vi "Create Segmented Mask.vi"(0 "Specification Cluster":cluster{"X":dbl[], "Y":dbl[]}[](array[cluster]) {"Y" format="%.2p"; "X" format="%.2p"}, 1 "dx":dbl format="%.2p", 2 "x0":dbl=1.0 format="%.2p", 3 "error in (no error)":errorcluster, 4 "Reset":bool) -> (5 "Limit":cluster{"x0":dbl, "dx":dbl, "Y":dbl[]} {"Y" format="%.2p"; "dx" format="%.2p"; "x0" format="%.2p"}, 6 "error out":errorcluster)   [LabVIEW 2020, in "NI_MAPro.lvlib"]
doc: "Creates continuous or segmented masks in the time domain or in the frequency domain. You can use different instances of this VI to create multiple limits. Wire data to the <B>Specification Cluster</B> input to determine the polymorphic instance to use or manually select the instance."
uses:
  NI_MAPro.lvlib
  NI_MABase.lvlib
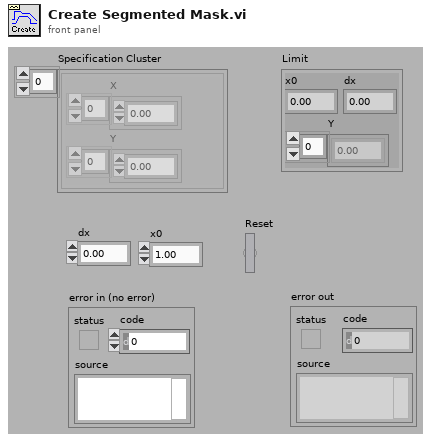
[diagram p1: front panel]
types:
  T1 = cluster{"x0":dbl, "dx":dbl, "Array Constant":dbl[]}
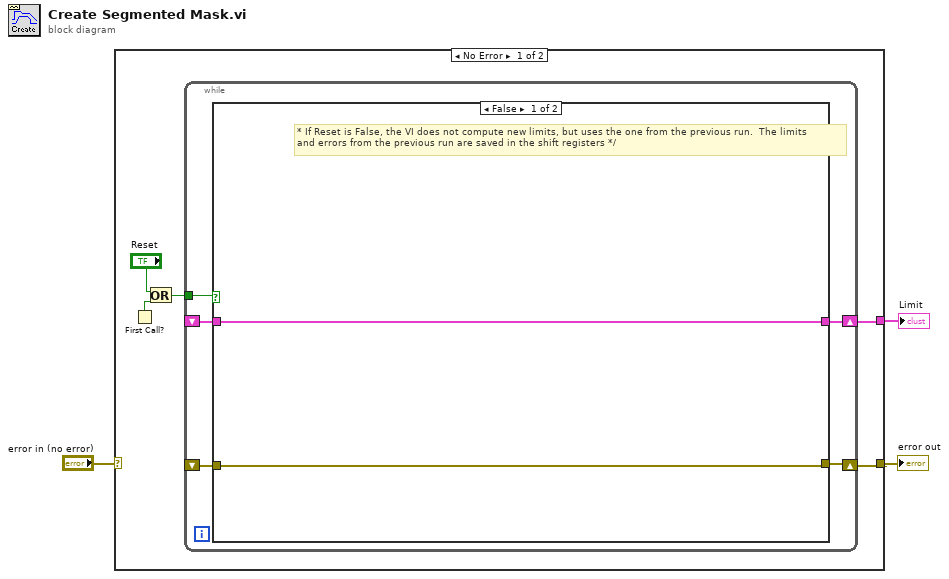
[diagram p0: block diagram]
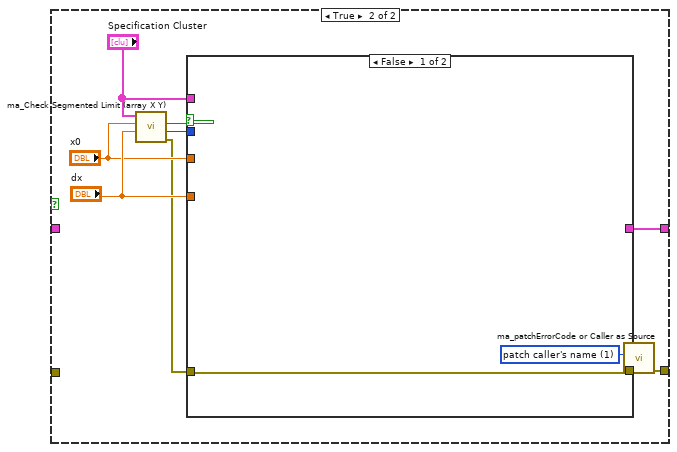
[diagram p2: hidden frame]
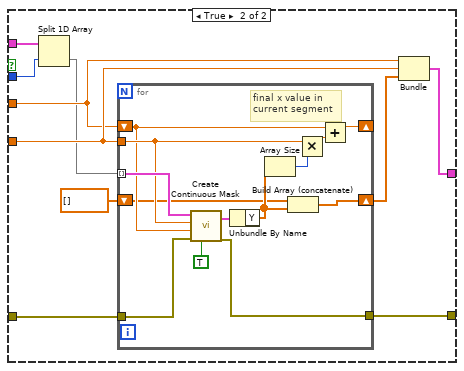
[diagram p3: hidden frame]
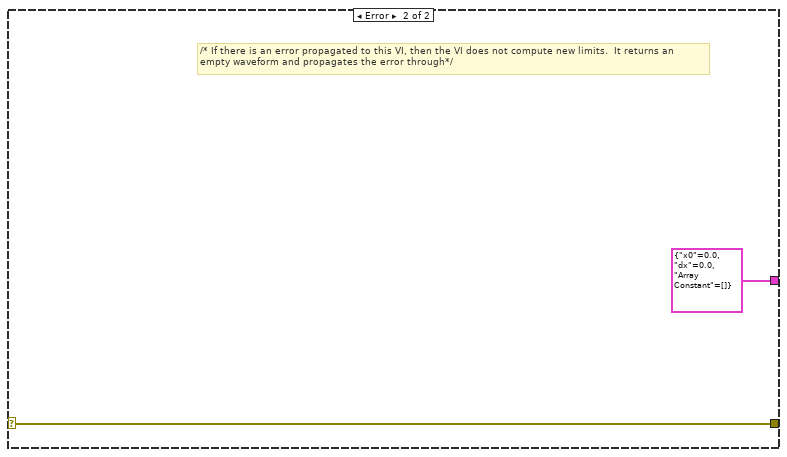
[diagram p4: hidden frame]
diagram:
  n1 = case shown="No Error" "error in (no error)" {
    selector: "error in (no error)" -> [_ w53]
    tunnel: [w8 w53] -> w3
    tunnel: [w4 T1 {"x0"=0.0, "dx"=0.0, "Array Constant"=[]}] -> w2
    frame No Error {
      n2 = First Call?() -> (First Call?: T/F=w6:bool)
      n3 = Or(x="Reset", y=w6) -> (x .or. y?=w5:bool)
      n4 = while {
        tunnel: w5 -> [w9]
        shift-left: _ -> [w10]
        shift-right: [w14] -> w8
        shift-left: _ -> [w11]
        shift-right: [w13] -> w4
        stop <- FALSE continue-if-true
        n5 = case shown="False" w9 {
          tunnel: [w16 w24] -> w13
          tunnel: [w15 w23] -> w14
          tunnel: w11 -> [w16 _]
          tunnel: w10 -> [w15 _]
          frame False {
            # "* If Reset is False, the VI does not compute new limits, but uses the one from the previous run.  The limits\nand errors from the previous run are saved in the shift registers */"
          }
          frame True {
            n6 = call "ma_Check Segmented Limit (array X Y).vi"("Specification Cluster"="Specification Cluster", "x0"="x0", "dx"="dx") -> ("limit spec ok"=w19:bool, "1st valid segment index"=w17:i32, "error out"=w18:errorcluster)  [unwired: 5 in]
            n7 = case shown="False" w19 {
              tunnel: "dx" -> [_ w35]
              tunnel: w18 -> [w25 w37]
              tunnel: [w26 w36] -> w23
              tunnel: [T1 {"x0"=0.0, "dx"=0.0, "Array Constant"=[]} w29] -> w24
              tunnel: "Specification Cluster" -> [_ w32]
              tunnel: "x0" -> [_ w33]
              tunnel: w17 -> [_ w31]
              frame False {
                w27 = u16 1 items=["patch error code", "patch caller's name"] ("operation")
                n8 = call "ma_patchErrorCode or Caller as Source.vi"("error in (no error)"=w25, "operation"=w27) -> ("error out"=w26:errorcluster)  [unwired: 2 in, 7 out]
              }
              frame True {
                n9 = Split 1D Array(array=w32, index=w31) -> (second subarray=w30:cluster{"X":dbl[], "Y":dbl[]}[])  [unwired: 1 out]
                n10 = for {
                  tunnel: w30 -> [w48] mode=indexing
                  shift-right: [w41] -> _
                  shift-left: w33 -> [w40]
                  shift-right: [w51] -> w34
                  shift-left: dbl[] [] ("Array Constant") -> [w39]
                  tunnel: w35 -> [w44]
                  tunnel: w37 -> [w50]
                  tunnel: [w49] -> w36
                  # "final x value in\ncurrent segment"
                  n11 = call "Create Continuous Mask.vi"("Specification Cluster"=w48, "dx"=w44, "x0"=w40, "error in (no error)"=w50, "Reset"=TRUE) -> ("Limit"=w46:cluster{"x0":dbl, "dx":dbl, "Y":dbl[]}, "error out"=w49:errorcluster)
                  n12 = Unbundle By Name(w46) -> ("Y"=w43:dbl[])
                  n13 = Array Size(array=w43) -> (size(s)=w45:i32)
                  n14 = Build Array (concatenate)(w39, w43) -> (w51:dbl[])
                  n15 = Multiply(x=w45, y=w44) -> (x*y=w42:dbl)
                  n16 = Add(x=w40, y=w42) -> (x+y=w41:dbl)
                }
                n17 = Bundle("x0"=w33, "dx"=w35, "Array Constant"=w34) -> (w29:T1)  [unwired: 1 out]
              }
            }
          }
        }
      }
    }
    frame Error {
      # "/* If there is an error propagated to this VI, then the VI does not compute new limits.  It returns an\nempty waveform and propagates the error through*/"
    }
  }
  "error out" <- w3
  "Limit" <- w2
